vi "Autonomous2Independent.vi"() -> ()   [LabVIEW 2017]
doc: "This VI is called when autonomous begins, and will automatically be terminated when autonomous ends. You can carry out timed or sensor driven robot movement independently without needing to return to the caller."
uses:
  <vilib>/Rock Robotics/WPI/DriverStation/WPI_DriverStationPositionInfo.ctl
  <vilib>/Rock Robotics/WPI/Utilities/WPI_GetSetVariantRefNum.vi
panel:
  out "Distance 32":dbl
  out "Distance 31":dbl
  out "Distance 30":dbl
  out "Distance 29":dbl
  out "Distance 28":dbl
  out "Distance 27":dbl
  out "Distance 26":dbl
  out "Distance 25":dbl
  out "Distance 24":dbl
  out "Distance 23":dbl
  out "Distance 22":dbl
  out "Distance 21":dbl
  out "Distance 20":dbl
  out "Distance 19":dbl
  out "Distance 18":dbl
  out "Distance 17":dbl
  out "Distance 16":dbl
  out "Distance 15":dbl
  out "Distance 14":dbl
  out "Distance 13":dbl
  out "Distance 12":dbl
  out "Distance 11":dbl
  out "Distance 10":dbl
  out "Distance 9":dbl
  out "Distance 6":dbl
  out "Distance 5":dbl
  out "Distance":dbl
  out "Distance 2":dbl
  out "substring":string
  out "Position":T1
  # "Be sure to right-click and choose Data Operations>>Make Current Value default if you want to save the array values with the VI"
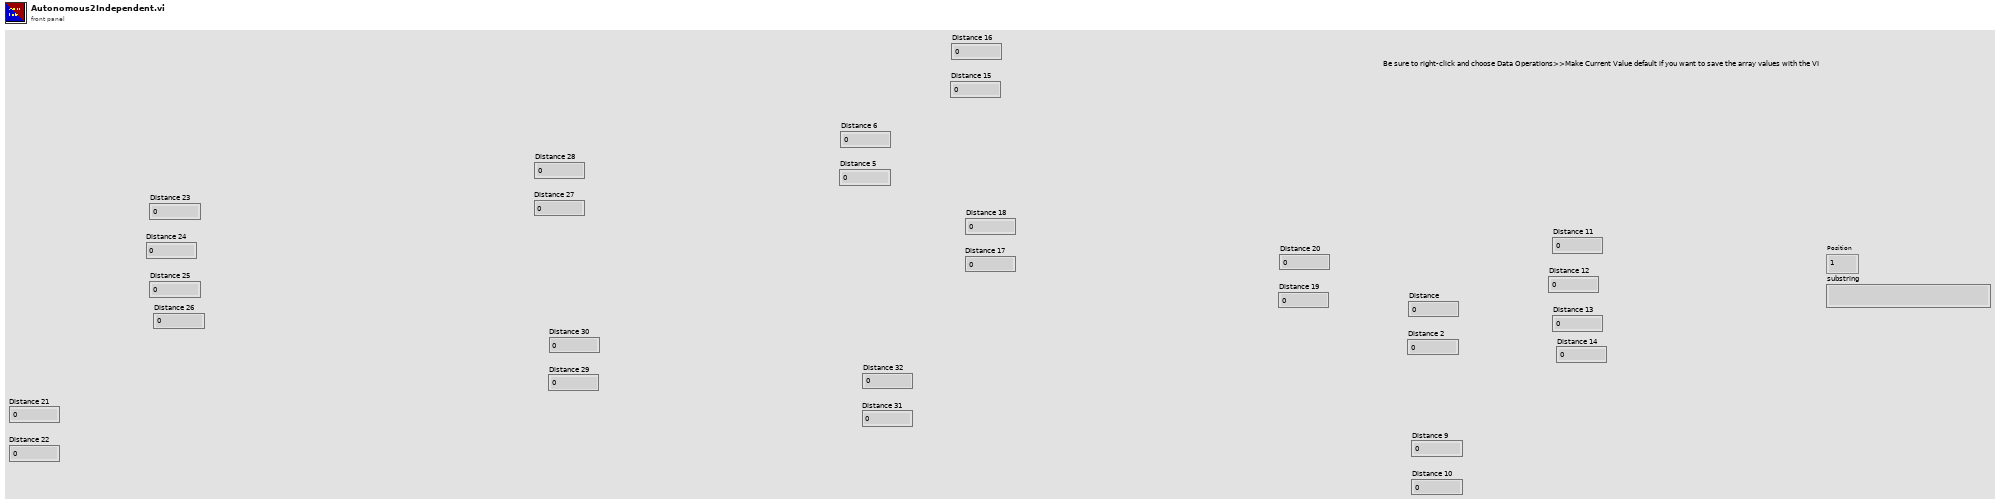
[diagram p1: front panel]
types:
  T1 = typedef "WPI_DriverStationPositionInfo.ctl" = enum16{"1", "2", "3"}
  T2 = typedef "WPI_EncoderDevRef.ctl" = cluster{"DevStatus":errorcluster, "EncoderIndex":T3, "CounterIndex":T4, "DistancePerCount":dbl, "Decoding Type":T5}
  T3 = typedef "FPGA_EncoderIdx.ctl" = enum8{"Enc 0", "Enc 1", "Enc 2", "Enc 3", "Enc 4", "Enc 5", "Enc 6", "Enc 7", "Invalid"}
  T4 = typedef "FPGA_CounterCtrSystemIndex.ctl" = enum8{"Ctr 0", "Ctr 1", "Ctr 2", "Ctr 3", "Ctr 4", "Ctr 5", "Ctr 6", "Ctr 7", "Invalid"}
  T5 = typedef "WPI_EncoderType.ctl" = enum16{"1x", "2x", "4x"}
  T6 = typedef "WPI_RobotDriveDevRef.ctl" = cluster{"DevStatus":errorcluster, "Motors[]":T7[], "Square Inputs":bool, "Max Output":dbl}
  T7 = typedef "WPI_MotorControlDeviceRef.ctl" = cluster{"DeviceStatus":errorcluster, "Type":T8, "PWM":cluster{"PWM Channel":T9, "DeadBand":T10}, "CAN":cluster{"Device Number":u8, "SetOutput VI Ref":variant, "GetOutput VI Ref":variant, "Enable VI Ref":variant, "Disable VI Ref":variant, "Data":variant}, "Invert":bool, "DIO PWM":cluster{"PWM \"Enable\" Channel":T9, "DIOChannel":T11, "PWM Rate":dbl}}
  T8 = typedef "WPI_MotorControlType.ctl" = enum16{"PWM", "CAN", "DIO PWM"}
  T9 = typedef "FPGA_DIOPWMChannel.ctl" = enum8{"PWM 0", "PWM 1", "PWM 2", "PWM 3", "PWM 4", "PWM 5", "PWM 6", "PWM 7", "PWM 8", "PWM 9", "PWM MXP 0", "PWM MXP 1", "PWM MXP 2", "PWM MXP 3", "PWM MXP 4", "PWM MXP 5", "PWM MXP 6", "PWM MXP 7", "PWM MXP 8", "PWM MXP 9", "Invalid"}
  T10 = typedef "WPI_PWMDeadband.ctl" = cluster{"Name":string, "maxPositivePwm":i32, "minPositivePwm":i32, "centerPwm":i32, "maxNegativePwm":i32, "minNegativePwm":i32, "angularRange":u16}
  T11 = typedef "FPGA_DIOChannel.ctl" = enum8{"DIO 0", "DIO 1", "DIO 2", "DIO 3", "DIO 4", "DIO 5", "DIO 6", "DIO 7", "DIO 8", "DIO 9", "DIO MXP 0", "DIO MXP 1", "DIO MXP 2", "DIO MXP 3", "DIO MXP 4", "DIO MXP 5", "DIO MXP 6", "DIO MXP 7", "DIO MXP 8", "DIO MXP 9", "DIO MXP 10", "DIO MXP 11", "DIO MXP 12", "DIO MXP 13", "DIO MXP 14", "DIO MXP 15", "SPI Port CS1", "SPI Port CS2", "SPI Port CS3", "SPI Port MISO", "SPI Port MOSI", "Invalid"}
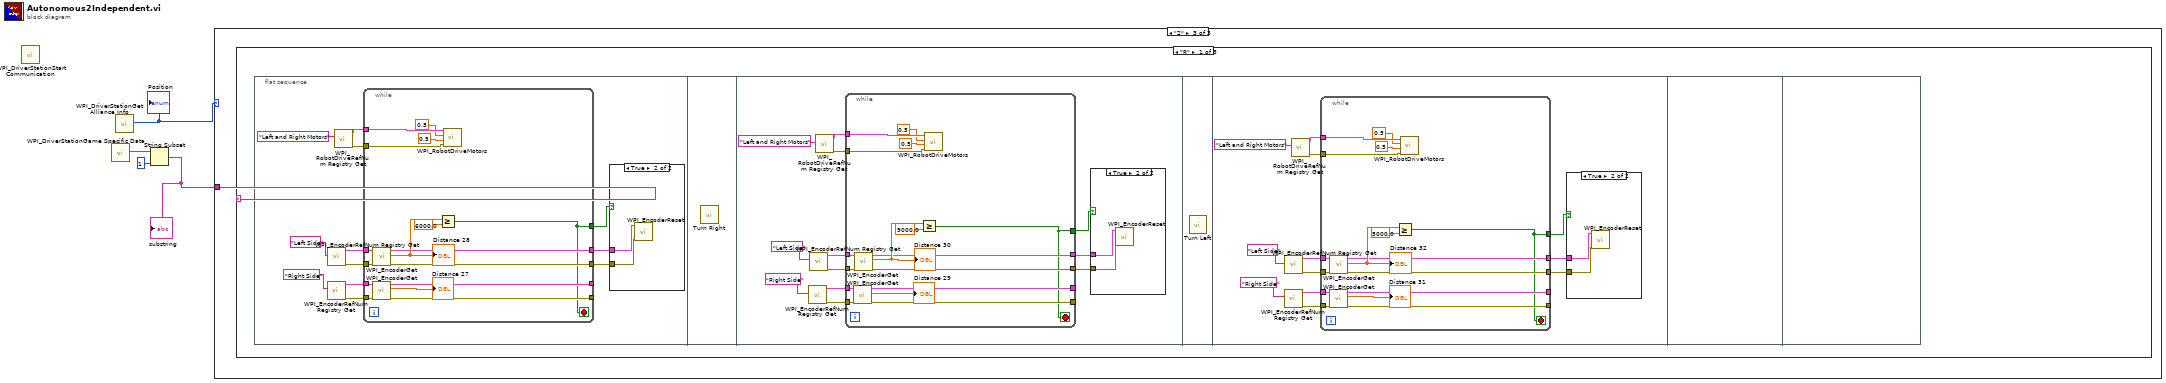
[diagram p0: block diagram]
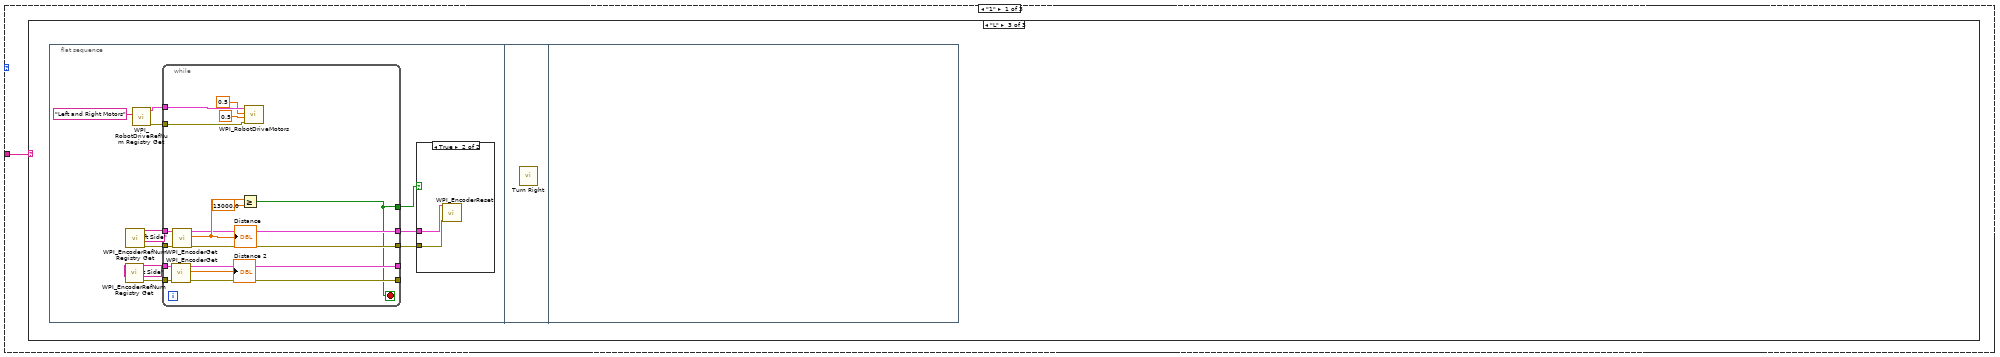
[diagram p2: hidden frame]
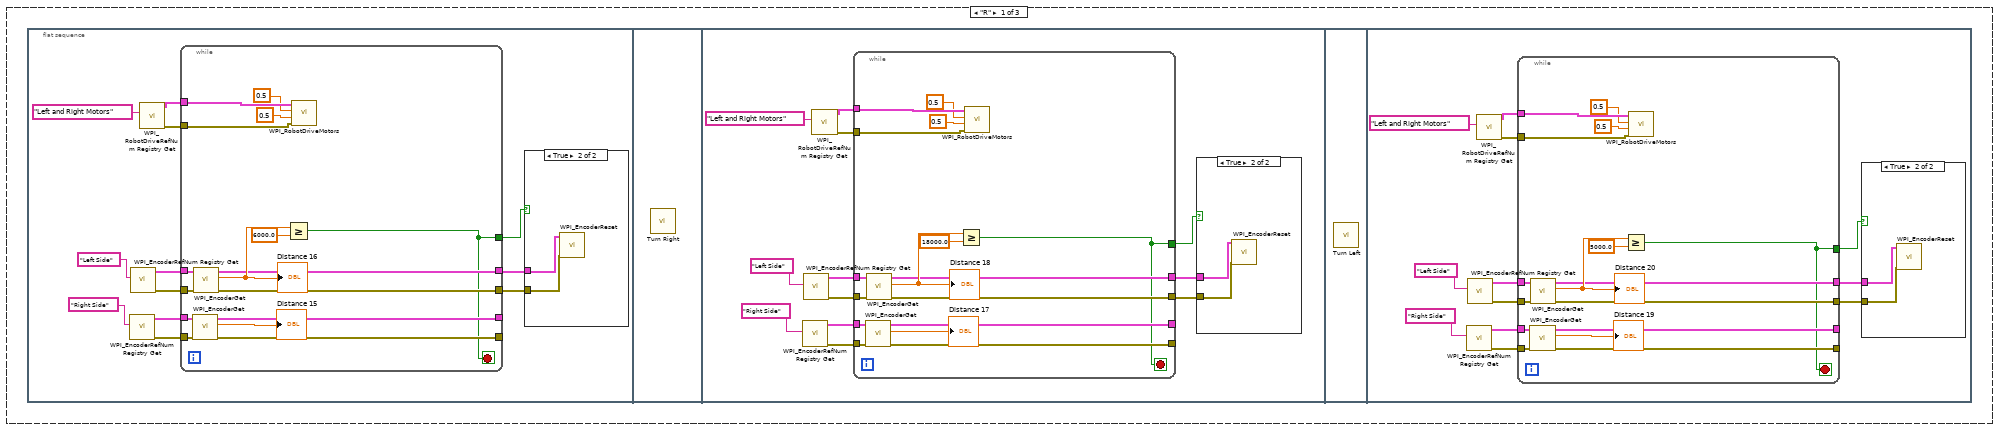
[diagram p3: hidden frame]
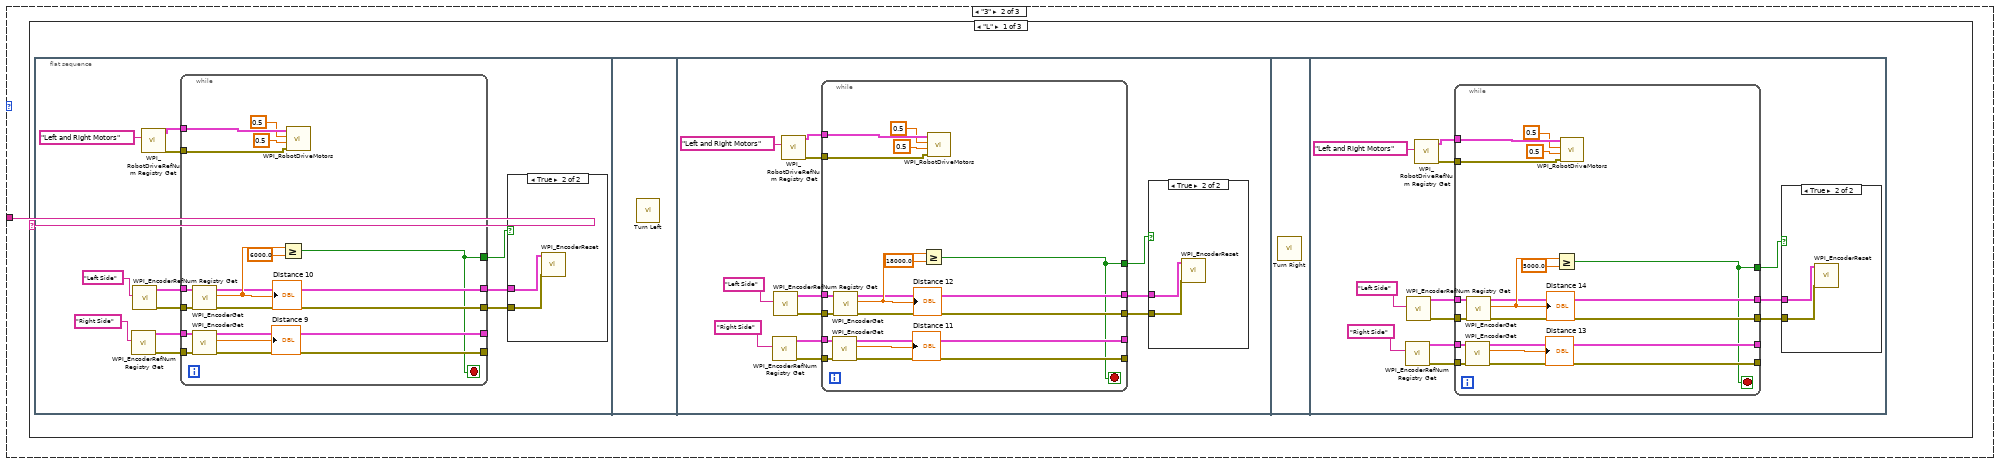
[diagram p9: hidden frame]
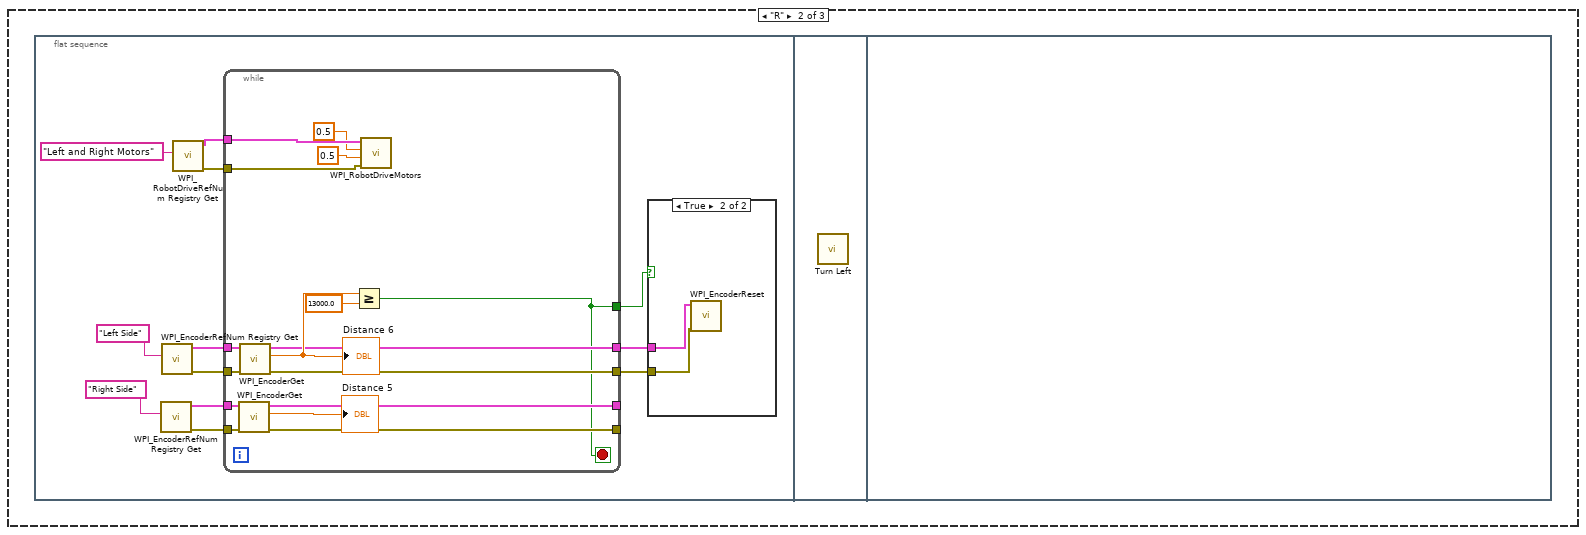
[diagram p13: hidden frame]
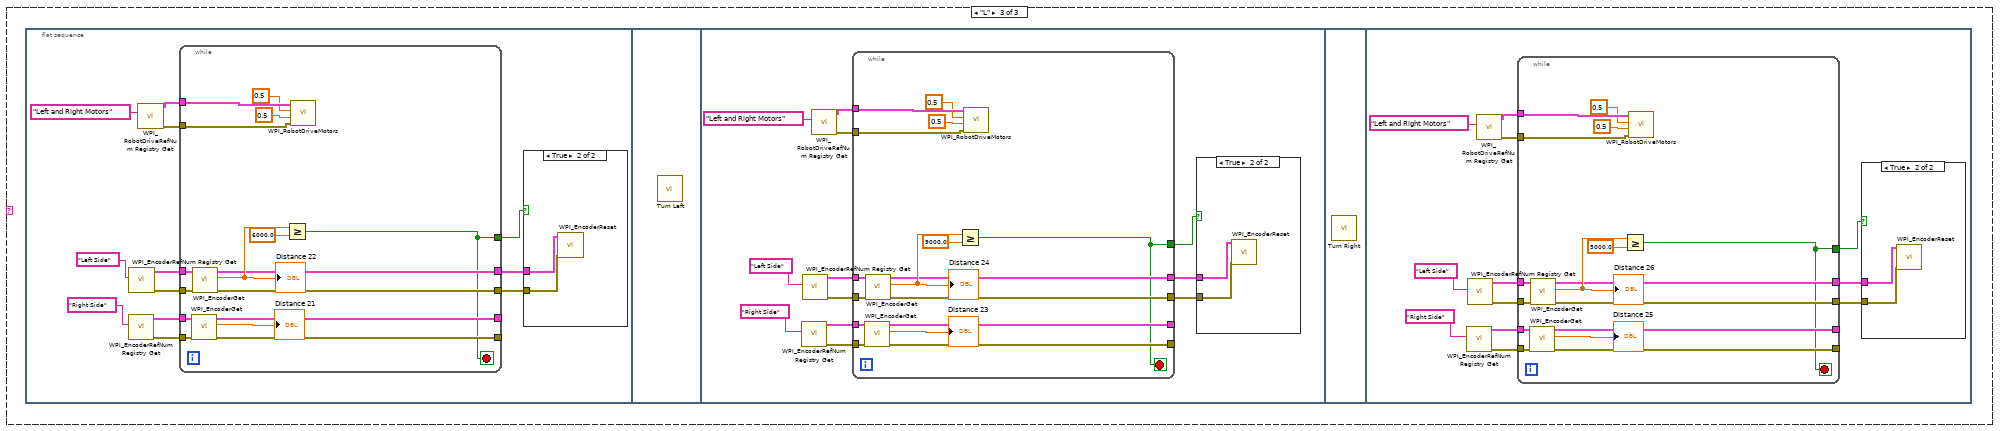
[diagram p20: hidden frame]
diagram:
  n1 = call <vilib>:"WPI_DriverStationStart Communication.vi"() -> ()  [unwired: 12 in]
  n2 = call <vilib>:"WPI_DriverStationGame Specific Data.vi"() -> ("Game Specific Data"=w4:string)  [unwired: 11 in]
  n3 = call <vilib>:"WPI_DriverStationGet Alliance Info.vi"() -> ("Position"=w2:T1)  [unwired: 6 in, 5 out]
  "Position" <- w2
  n4 = String Subset(string=w4, length (rest)=1 ("length (rest)")) -> (substring=w1:string)  [unwired: 1 in]
  "substring" <- w1
  n5 = case shown="\"2\"" w2 {
    tunnel: w1 -> [w5 w126 w247]
    frame "1" {
      n6 = case shown="\"L\"" w5 {
        frame "R" {
          n7 = flat-sequence {
            frame #0 {
              n8 = call <vilib>:"WPI_EncoderRefNum Registry Get.vi"("refnum name"="Right Side") -> ("error out"=w11:errorcluster, "EncoderDevRef"=w12:T2)  [unwired: 9 in]
              n9 = call <vilib>:"WPI_EncoderRefNum Registry Get.vi"("refnum name"="Left Side") -> ("error out"=w10:errorcluster, "EncoderDevRef"=w9:T2)  [unwired: 9 in]
              n10 = call <vilib>:"WPI_RobotDriveRefNum Registry Get.vi"("refnum name"="Left and Right Motors") -> ("error out"=w17:errorcluster, "RobotDriveDevRef"=w16:T6)  [unwired: 9 in]
              n11 = while {
                tunnel: w9 -> [w35]
                tunnel: w10 -> [w34]
                tunnel: w12 -> [w31]
                tunnel: w11 -> [w32]
                tunnel: [w28] -> w14
                tunnel: [w27] -> w15
                tunnel: [w26] -> _
                tunnel: [w25] -> _
                tunnel: [w24] -> w13
                tunnel: w16 -> [w23]
                tunnel: w17 -> [w22]
                stop <- w24 stop-if-true
                n12 = call <vilib>:"WPI_EncoderGet.vi"("error in (no error)"=w32, "EncoderDevRef"=w31) -> ("error out"=w25:errorcluster, "Distance"=→"Distance 15":dbl, "EncoderDevRef"=w26:T2)  [unwired: 4 in, 3 out]
                n13 = call <vilib>:"WPI_EncoderGet.vi"("error in (no error)"=w34, "EncoderDevRef"=w35) -> ("error out"=w27:errorcluster, "Distance"=w30:dbl, "EncoderDevRef"=w28:T2)  [unwired: 4 in, 3 out]
                "Distance 16" <- w30
                n14 = Greater Or Equal?(x=w30, y=6000.0) -> (x >= y?=w24:bool)
                n15 = call <vilib>:"WPI_RobotDriveMotors.vi"("error in (no error)"=w22, "RightSpeed"=0.5, "LeftSpeed"=0.5, "RobotDriveDevRef"=w23) -> ()  [unwired: 5 in, 3 out]
              }
              n16 = case shown="True" w13 {
                tunnel: w14 -> [_ w19]
                tunnel: w15 -> [_ w18]
                frame False {
                }
                frame True {
                  n17 = call <vilib>:"WPI_EncoderReset.vi"("error in (no error)"=w18, "EncoderDevRef"=w19) -> ()  [unwired: 8 in, 2 out]
                }
              }
            }
            frame #1 {
              n18 = call "Turn Right.vi"() -> ()  [unwired: 12 in]
            }
            frame #2 {
              n19 = call <vilib>:"WPI_EncoderRefNum Registry Get.vi"("refnum name"="Right Side") -> ("error out"=w45:errorcluster, "EncoderDevRef"=w44:T2)  [unwired: 9 in]
              n20 = call <vilib>:"WPI_EncoderRefNum Registry Get.vi"("refnum name"="Left Side") -> ("error out"=w46:errorcluster, "EncoderDevRef"=w47:T2)  [unwired: 9 in]
              n21 = call <vilib>:"WPI_RobotDriveRefNum Registry Get.vi"("refnum name"="Left and Right Motors") -> ("error out"=w36:errorcluster, "RobotDriveDevRef"=w37:T6)  [unwired: 9 in]
              n22 = while {
                tunnel: w47 -> [w65]
                tunnel: w46 -> [w64]
                tunnel: w44 -> [w61]
                tunnel: w45 -> [w62]
                tunnel: [w58] -> w40
                tunnel: [w57] -> w39
                tunnel: [w56] -> _
                tunnel: [w55] -> _
                tunnel: [w54] -> w41
                tunnel: w37 -> [w53]
                tunnel: w36 -> [w52]
                stop <- w54 stop-if-true
                n23 = call <vilib>:"WPI_EncoderGet.vi"("error in (no error)"=w62, "EncoderDevRef"=w61) -> ("error out"=w55:errorcluster, "Distance"=→"Distance 17":dbl, "EncoderDevRef"=w56:T2)  [unwired: 4 in, 3 out]
                n24 = call <vilib>:"WPI_EncoderGet.vi"("error in (no error)"=w64, "EncoderDevRef"=w65) -> ("error out"=w57:errorcluster, "Distance"=w60:dbl, "EncoderDevRef"=w58:T2)  [unwired: 4 in, 3 out]
                "Distance 18" <- w60
                n25 = Greater Or Equal?(x=w60, y=18000.0) -> (x >= y?=w54:bool)
                n26 = call <vilib>:"WPI_RobotDriveMotors.vi"("error in (no error)"=w52, "RightSpeed"=0.5, "LeftSpeed"=0.5, "RobotDriveDevRef"=w53) -> ()  [unwired: 5 in, 3 out]
              }
              n27 = case shown="True" w41 {
                tunnel: w40 -> [_ w49]
                tunnel: w39 -> [_ w48]
                frame False {
                }
                frame True {
                  n28 = call <vilib>:"WPI_EncoderReset.vi"("error in (no error)"=w48, "EncoderDevRef"=w49) -> ()  [unwired: 8 in, 2 out]
                }
              }
            }
            frame #3 {
              n29 = call "Turn Left.vi"() -> ()  [unwired: 12 in]
            }
            frame #4 {
              n30 = call <vilib>:"WPI_EncoderRefNum Registry Get.vi"("refnum name"="Right Side") -> ("error out"=w75:errorcluster, "EncoderDevRef"=w74:T2)  [unwired: 9 in]
              n31 = call <vilib>:"WPI_EncoderRefNum Registry Get.vi"("refnum name"="Left Side") -> ("error out"=w76:errorcluster, "EncoderDevRef"=w77:T2)  [unwired: 9 in]
              n32 = call <vilib>:"WPI_RobotDriveRefNum Registry Get.vi"("refnum name"="Left and Right Motors") -> ("error out"=w66:errorcluster, "RobotDriveDevRef"=w67:T6)  [unwired: 9 in]
              n33 = while {
                tunnel: w77 -> [w95]
                tunnel: w76 -> [w94]
                tunnel: w74 -> [w91]
                tunnel: w75 -> [w92]
                tunnel: [w88] -> w70
                tunnel: [w87] -> w69
                tunnel: [w86] -> _
                tunnel: [w85] -> _
                tunnel: [w84] -> w71
                tunnel: w67 -> [w83]
                tunnel: w66 -> [w82]
                stop <- w84 stop-if-true
                n34 = call <vilib>:"WPI_EncoderGet.vi"("error in (no error)"=w92, "EncoderDevRef"=w91) -> ("error out"=w85:errorcluster, "Distance"=→"Distance 19":dbl, "EncoderDevRef"=w86:T2)  [unwired: 4 in, 3 out]
                n35 = call <vilib>:"WPI_EncoderGet.vi"("error in (no error)"=w94, "EncoderDevRef"=w95) -> ("error out"=w87:errorcluster, "Distance"=w90:dbl, "EncoderDevRef"=w88:T2)  [unwired: 4 in, 3 out]
                "Distance 20" <- w90
                n36 = Greater Or Equal?(x=w90, y=5000.0) -> (x >= y?=w84:bool)
                n37 = call <vilib>:"WPI_RobotDriveMotors.vi"("error in (no error)"=w82, "RightSpeed"=0.5, "LeftSpeed"=0.5, "RobotDriveDevRef"=w83) -> ()  [unwired: 5 in, 3 out]
              }
              n38 = case shown="True" w71 {
                tunnel: w70 -> [_ w79]
                tunnel: w69 -> [_ w78]
                frame False {
                }
                frame True {
                  n39 = call <vilib>:"WPI_EncoderReset.vi"("error in (no error)"=w78, "EncoderDevRef"=w79) -> ()  [unwired: 8 in, 2 out]
                }
              }
            }
          }
        }
        frame Default {
        }
        frame "L" {
          n40 = flat-sequence {
            frame #0 {
              n41 = call <vilib>:"WPI_EncoderRefNum Registry Get.vi"("refnum name"="Right Side") -> ("error out"=w105:errorcluster, "EncoderDevRef"=w104:T2)  [unwired: 9 in]
              n42 = call <vilib>:"WPI_EncoderRefNum Registry Get.vi"("refnum name"="Left Side") -> ("error out"=w106:errorcluster, "EncoderDevRef"=w107:T2)  [unwired: 9 in]
              n43 = call <vilib>:"WPI_RobotDriveRefNum Registry Get.vi"("refnum name"="Left and Right Motors") -> ("error out"=w96:errorcluster, "RobotDriveDevRef"=w97:T6)  [unwired: 9 in]
              n44 = while {
                tunnel: w107 -> [w125]
                tunnel: w106 -> [w124]
                tunnel: w104 -> [w121]
                tunnel: w105 -> [w122]
                tunnel: [w118] -> w100
                tunnel: [w117] -> w99
                tunnel: [w116] -> _
                tunnel: [w115] -> _
                tunnel: [w114] -> w101
                tunnel: w97 -> [w113]
                tunnel: w96 -> [w112]
                stop <- w114 stop-if-true
                n45 = call <vilib>:"WPI_EncoderGet.vi"("error in (no error)"=w122, "EncoderDevRef"=w121) -> ("error out"=w115:errorcluster, "Distance"=→"Distance 2":dbl, "EncoderDevRef"=w116:T2)  [unwired: 4 in, 3 out]
                n46 = call <vilib>:"WPI_EncoderGet.vi"("error in (no error)"=w124, "EncoderDevRef"=w125) -> ("error out"=w117:errorcluster, "Distance"=w120:dbl, "EncoderDevRef"=w118:T2)  [unwired: 4 in, 3 out]
                "Distance" <- w120
                n47 = Greater Or Equal?(x=w120, y=13000.0) -> (x >= y?=w114:bool)
                n48 = call <vilib>:"WPI_RobotDriveMotors.vi"("error in (no error)"=w112, "RightSpeed"=0.5, "LeftSpeed"=0.5, "RobotDriveDevRef"=w113) -> ()  [unwired: 5 in, 3 out]
              }
              n49 = case shown="True" w101 {
                tunnel: w100 -> [_ w109]
                tunnel: w99 -> [_ w108]
                frame False {
                }
                frame True {
                  n50 = call <vilib>:"WPI_EncoderReset.vi"("error in (no error)"=w108, "EncoderDevRef"=w109) -> ()  [unwired: 8 in, 2 out]
                }
              }
            }
            frame #1 {
              n51 = call "Turn Right.vi"() -> ()  [unwired: 12 in]
            }
            frame #2 {
            }
          }
        }
      }
    }
    frame "3" {
      n52 = case shown="\"L\"" w126 {
        frame "L" {
          n53 = flat-sequence {
            frame #0 {
              n54 = call <vilib>:"WPI_EncoderRefNum Registry Get.vi"("refnum name"="Right Side") -> ("error out"=w132:errorcluster, "EncoderDevRef"=w133:T2)  [unwired: 9 in]
              n55 = call <vilib>:"WPI_EncoderRefNum Registry Get.vi"("refnum name"="Left Side") -> ("error out"=w131:errorcluster, "EncoderDevRef"=w130:T2)  [unwired: 9 in]
              n56 = call <vilib>:"WPI_RobotDriveRefNum Registry Get.vi"("refnum name"="Left and Right Motors") -> ("error out"=w138:errorcluster, "RobotDriveDevRef"=w137:T6)  [unwired: 9 in]
              n57 = while {
                tunnel: w130 -> [w156]
                tunnel: w131 -> [w155]
                tunnel: w133 -> [w152]
                tunnel: w132 -> [w153]
                tunnel: [w149] -> w135
                tunnel: [w148] -> w136
                tunnel: [w147] -> _
                tunnel: [w146] -> _
                tunnel: [w145] -> w134
                tunnel: w137 -> [w144]
                tunnel: w138 -> [w143]
                stop <- w145 stop-if-true
                n58 = call <vilib>:"WPI_EncoderGet.vi"("error in (no error)"=w153, "EncoderDevRef"=w152) -> ("error out"=w146:errorcluster, "Distance"=→"Distance 9":dbl, "EncoderDevRef"=w147:T2)  [unwired: 4 in, 3 out]
                n59 = call <vilib>:"WPI_EncoderGet.vi"("error in (no error)"=w155, "EncoderDevRef"=w156) -> ("error out"=w148:errorcluster, "Distance"=w151:dbl, "EncoderDevRef"=w149:T2)  [unwired: 4 in, 3 out]
                "Distance 10" <- w151
                n60 = Greater Or Equal?(x=w151, y=6000.0) -> (x >= y?=w145:bool)
                n61 = call <vilib>:"WPI_RobotDriveMotors.vi"("error in (no error)"=w143, "RightSpeed"=0.5, "LeftSpeed"=0.5, "RobotDriveDevRef"=w144) -> ()  [unwired: 5 in, 3 out]
              }
              n62 = case shown="True" w134 {
                tunnel: w135 -> [_ w140]
                tunnel: w136 -> [_ w139]
                frame False {
                }
                frame True {
                  n63 = call <vilib>:"WPI_EncoderReset.vi"("error in (no error)"=w139, "EncoderDevRef"=w140) -> ()  [unwired: 8 in, 2 out]
                }
              }
            }
            frame #1 {
              n64 = call "Turn Left.vi"() -> ()  [unwired: 12 in]
            }
            frame #2 {
              n65 = call <vilib>:"WPI_EncoderRefNum Registry Get.vi"("refnum name"="Right Side") -> ("error out"=w166:errorcluster, "EncoderDevRef"=w165:T2)  [unwired: 9 in]
              n66 = call <vilib>:"WPI_EncoderRefNum Registry Get.vi"("refnum name"="Left Side") -> ("error out"=w167:errorcluster, "EncoderDevRef"=w168:T2)  [unwired: 9 in]
              n67 = call <vilib>:"WPI_RobotDriveRefNum Registry Get.vi"("refnum name"="Left and Right Motors") -> ("error out"=w157:errorcluster, "RobotDriveDevRef"=w158:T6)  [unwired: 9 in]
              n68 = while {
                tunnel: w168 -> [w186]
                tunnel: w167 -> [w185]
                tunnel: w165 -> [w182]
                tunnel: w166 -> [w183]
                tunnel: [w179] -> w161
                tunnel: [w178] -> w160
                tunnel: [w177] -> _
                tunnel: [w176] -> _
                tunnel: [w175] -> w162
                tunnel: w158 -> [w174]
                tunnel: w157 -> [w173]
                stop <- w175 stop-if-true
                n69 = call <vilib>:"WPI_EncoderGet.vi"("error in (no error)"=w183, "EncoderDevRef"=w182) -> ("error out"=w176:errorcluster, "Distance"=→"Distance 11":dbl, "EncoderDevRef"=w177:T2)  [unwired: 4 in, 3 out]
                n70 = call <vilib>:"WPI_EncoderGet.vi"("error in (no error)"=w185, "EncoderDevRef"=w186) -> ("error out"=w178:errorcluster, "Distance"=w181:dbl, "EncoderDevRef"=w179:T2)  [unwired: 4 in, 3 out]
                "Distance 12" <- w181
                n71 = Greater Or Equal?(x=w181, y=18000.0) -> (x >= y?=w175:bool)
                n72 = call <vilib>:"WPI_RobotDriveMotors.vi"("error in (no error)"=w173, "RightSpeed"=0.5, "LeftSpeed"=0.5, "RobotDriveDevRef"=w174) -> ()  [unwired: 5 in, 3 out]
              }
              n73 = case shown="True" w162 {
                tunnel: w161 -> [_ w170]
                tunnel: w160 -> [_ w169]
                frame False {
                }
                frame True {
                  n74 = call <vilib>:"WPI_EncoderReset.vi"("error in (no error)"=w169, "EncoderDevRef"=w170) -> ()  [unwired: 8 in, 2 out]
                }
              }
            }
            frame #3 {
              n75 = call "Turn Right.vi"() -> ()  [unwired: 12 in]
            }
            frame #4 {
              n76 = call <vilib>:"WPI_EncoderRefNum Registry Get.vi"("refnum name"="Right Side") -> ("error out"=w196:errorcluster, "EncoderDevRef"=w195:T2)  [unwired: 9 in]
              n77 = call <vilib>:"WPI_EncoderRefNum Registry Get.vi"("refnum name"="Left Side") -> ("error out"=w197:errorcluster, "EncoderDevRef"=w198:T2)  [unwired: 9 in]
              n78 = call <vilib>:"WPI_RobotDriveRefNum Registry Get.vi"("refnum name"="Left and Right Motors") -> ("error out"=w187:errorcluster, "RobotDriveDevRef"=w188:T6)  [unwired: 9 in]
              n79 = while {
                tunnel: w198 -> [w216]
                tunnel: w197 -> [w215]
                tunnel: w195 -> [w212]
                tunnel: w196 -> [w213]
                tunnel: [w209] -> w191
                tunnel: [w208] -> w190
                tunnel: [w207] -> _
                tunnel: [w206] -> _
                tunnel: [w205] -> w192
                tunnel: w188 -> [w204]
                tunnel: w187 -> [w203]
                stop <- w205 stop-if-true
                n80 = call <vilib>:"WPI_EncoderGet.vi"("error in (no error)"=w213, "EncoderDevRef"=w212) -> ("error out"=w206:errorcluster, "Distance"=→"Distance 13":dbl, "EncoderDevRef"=w207:T2)  [unwired: 4 in, 3 out]
                n81 = call <vilib>:"WPI_EncoderGet.vi"("error in (no error)"=w215, "EncoderDevRef"=w216) -> ("error out"=w208:errorcluster, "Distance"=w211:dbl, "EncoderDevRef"=w209:T2)  [unwired: 4 in, 3 out]
                "Distance 14" <- w211
                n82 = Greater Or Equal?(x=w211, y=5000.0) -> (x >= y?=w205:bool)
                n83 = call <vilib>:"WPI_RobotDriveMotors.vi"("error in (no error)"=w203, "RightSpeed"=0.5, "LeftSpeed"=0.5, "RobotDriveDevRef"=w204) -> ()  [unwired: 5 in, 3 out]
              }
              n84 = case shown="True" w192 {
                tunnel: w191 -> [_ w200]
                tunnel: w190 -> [_ w199]
                frame False {
                }
                frame True {
                  n85 = call <vilib>:"WPI_EncoderReset.vi"("error in (no error)"=w199, "EncoderDevRef"=w200) -> ()  [unwired: 8 in, 2 out]
                }
              }
            }
          }
        }
        frame "R" {
          n86 = flat-sequence {
            frame #0 {
              n87 = call <vilib>:"WPI_EncoderRefNum Registry Get.vi"("refnum name"="Right Side") -> ("error out"=w226:errorcluster, "EncoderDevRef"=w225:T2)  [unwired: 9 in]
              n88 = call <vilib>:"WPI_EncoderRefNum Registry Get.vi"("refnum name"="Left Side") -> ("error out"=w227:errorcluster, "EncoderDevRef"=w228:T2)  [unwired: 9 in]
              n89 = call <vilib>:"WPI_RobotDriveRefNum Registry Get.vi"("refnum name"="Left and Right Motors") -> ("error out"=w217:errorcluster, "RobotDriveDevRef"=w218:T6)  [unwired: 9 in]
              n90 = while {
                tunnel: w228 -> [w246]
                tunnel: w227 -> [w245]
                tunnel: w225 -> [w242]
                tunnel: w226 -> [w243]
                tunnel: [w239] -> w221
                tunnel: [w238] -> w220
                tunnel: [w237] -> _
                tunnel: [w236] -> _
                tunnel: [w235] -> w222
                tunnel: w218 -> [w234]
                tunnel: w217 -> [w233]
                stop <- w235 stop-if-true
                n91 = call <vilib>:"WPI_EncoderGet.vi"("error in (no error)"=w243, "EncoderDevRef"=w242) -> ("error out"=w236:errorcluster, "Distance"=→"Distance 5":dbl, "EncoderDevRef"=w237:T2)  [unwired: 4 in, 3 out]
                n92 = call <vilib>:"WPI_EncoderGet.vi"("error in (no error)"=w245, "EncoderDevRef"=w246) -> ("error out"=w238:errorcluster, "Distance"=w241:dbl, "EncoderDevRef"=w239:T2)  [unwired: 4 in, 3 out]
                "Distance 6" <- w241
                n93 = Greater Or Equal?(x=w241, y=13000.0) -> (x >= y?=w235:bool)
                n94 = call <vilib>:"WPI_RobotDriveMotors.vi"("error in (no error)"=w233, "RightSpeed"=0.5, "LeftSpeed"=0.5, "RobotDriveDevRef"=w234) -> ()  [unwired: 5 in, 3 out]
              }
              n95 = case shown="True" w222 {
                tunnel: w221 -> [_ w230]
                tunnel: w220 -> [_ w229]
                frame False {
                }
                frame True {
                  n96 = call <vilib>:"WPI_EncoderReset.vi"("error in (no error)"=w229, "EncoderDevRef"=w230) -> ()  [unwired: 8 in, 2 out]
                }
              }
            }
            frame #1 {
              n97 = call "Turn Left.vi"() -> ()  [unwired: 12 in]
            }
            frame #2 {
            }
          }
        }
        frame Default {
        }
      }
    }
    frame "2" {
      n98 = case shown="\"R\"" w247 {
        frame "R" {
          n99 = flat-sequence {
            frame #0 {
              n100 = call <vilib>:"WPI_EncoderRefNum Registry Get.vi"("refnum name"="Right Side") -> ("error out"=w253:errorcluster, "EncoderDevRef"=w254:T2)  [unwired: 9 in]
              n101 = call <vilib>:"WPI_EncoderRefNum Registry Get.vi"("refnum name"="Left Side") -> ("error out"=w252:errorcluster, "EncoderDevRef"=w251:T2)  [unwired: 9 in]
              n102 = call <vilib>:"WPI_RobotDriveRefNum Registry Get.vi"("refnum name"="Left and Right Motors") -> ("error out"=w259:errorcluster, "RobotDriveDevRef"=w258:T6)  [unwired: 9 in]
              n103 = while {
                tunnel: w251 -> [w277]
                tunnel: w252 -> [w276]
                tunnel: w254 -> [w273]
                tunnel: w253 -> [w274]
                tunnel: [w270] -> w256
                tunnel: [w269] -> w257
                tunnel: [w268] -> _
                tunnel: [w267] -> _
                tunnel: [w266] -> w255
                tunnel: w258 -> [w265]
                tunnel: w259 -> [w264]
                stop <- w266 stop-if-true
                n104 = call <vilib>:"WPI_EncoderGet.vi"("error in (no error)"=w274, "EncoderDevRef"=w273) -> ("error out"=w267:errorcluster, "Distance"=→"Distance 27":dbl, "EncoderDevRef"=w268:T2)  [unwired: 4 in, 3 out]
                n105 = call <vilib>:"WPI_EncoderGet.vi"("error in (no error)"=w276, "EncoderDevRef"=w277) -> ("error out"=w269:errorcluster, "Distance"=w272:dbl, "EncoderDevRef"=w270:T2)  [unwired: 4 in, 3 out]
                "Distance 28" <- w272
                n106 = Greater Or Equal?(x=w272, y=6000.0) -> (x >= y?=w266:bool)
                n107 = call <vilib>:"WPI_RobotDriveMotors.vi"("error in (no error)"=w264, "RightSpeed"=0.5, "LeftSpeed"=0.5, "RobotDriveDevRef"=w265) -> ()  [unwired: 5 in, 3 out]
              }
              n108 = case shown="True" w255 {
                tunnel: w256 -> [_ w261]
                tunnel: w257 -> [_ w260]
                frame False {
                }
                frame True {
                  n109 = call <vilib>:"WPI_EncoderReset.vi"("error in (no error)"=w260, "EncoderDevRef"=w261) -> ()  [unwired: 8 in, 2 out]
                }
              }
            }
            frame #1 {
              n110 = call "Turn Right.vi"() -> ()  [unwired: 12 in]
            }
            frame #2 {
              n111 = call <vilib>:"WPI_EncoderRefNum Registry Get.vi"("refnum name"="Right Side") -> ("error out"=w287:errorcluster, "EncoderDevRef"=w286:T2)  [unwired: 9 in]
              n112 = call <vilib>:"WPI_EncoderRefNum Registry Get.vi"("refnum name"="Left Side") -> ("error out"=w288:errorcluster, "EncoderDevRef"=w289:T2)  [unwired: 9 in]
              n113 = call <vilib>:"WPI_RobotDriveRefNum Registry Get.vi"("refnum name"="Left and Right Motors") -> ("error out"=w278:errorcluster, "RobotDriveDevRef"=w279:T6)  [unwired: 9 in]
              n114 = while {
                tunnel: w289 -> [w307]
                tunnel: w288 -> [w306]
                tunnel: w286 -> [w303]
                tunnel: w287 -> [w304]
                tunnel: [w300] -> w282
                tunnel: [w299] -> w281
                tunnel: [w298] -> _
                tunnel: [w297] -> _
                tunnel: [w296] -> w283
                tunnel: w279 -> [w295]
                tunnel: w278 -> [w294]
                stop <- w296 stop-if-true
                n115 = call <vilib>:"WPI_EncoderGet.vi"("error in (no error)"=w304, "EncoderDevRef"=w303) -> ("error out"=w297:errorcluster, "Distance"=→"Distance 29":dbl, "EncoderDevRef"=w298:T2)  [unwired: 4 in, 3 out]
                n116 = call <vilib>:"WPI_EncoderGet.vi"("error in (no error)"=w306, "EncoderDevRef"=w307) -> ("error out"=w299:errorcluster, "Distance"=w302:dbl, "EncoderDevRef"=w300:T2)  [unwired: 4 in, 3 out]
                "Distance 30" <- w302
                n117 = Greater Or Equal?(x=w302, y=9000.0) -> (x >= y?=w296:bool)
                n118 = call <vilib>:"WPI_RobotDriveMotors.vi"("error in (no error)"=w294, "RightSpeed"=0.5, "LeftSpeed"=0.5, "RobotDriveDevRef"=w295) -> ()  [unwired: 5 in, 3 out]
              }
              n119 = case shown="True" w283 {
                tunnel: w282 -> [_ w291]
                tunnel: w281 -> [_ w290]
                frame False {
                }
                frame True {
                  n120 = call <vilib>:"WPI_EncoderReset.vi"("error in (no error)"=w290, "EncoderDevRef"=w291) -> ()  [unwired: 8 in, 2 out]
                }
              }
            }
            frame #3 {
              n121 = call "Turn Left.vi"() -> ()  [unwired: 12 in]
            }
            frame #4 {
              n122 = call <vilib>:"WPI_EncoderRefNum Registry Get.vi"("refnum name"="Right Side") -> ("error out"=w317:errorcluster, "EncoderDevRef"=w316:T2)  [unwired: 9 in]
              n123 = call <vilib>:"WPI_EncoderRefNum Registry Get.vi"("refnum name"="Left Side") -> ("error out"=w318:errorcluster, "EncoderDevRef"=w319:T2)  [unwired: 9 in]
              n124 = call <vilib>:"WPI_RobotDriveRefNum Registry Get.vi"("refnum name"="Left and Right Motors") -> ("error out"=w308:errorcluster, "RobotDriveDevRef"=w309:T6)  [unwired: 9 in]
              n125 = while {
                tunnel: w319 -> [w337]
                tunnel: w318 -> [w336]
                tunnel: w316 -> [w333]
                tunnel: w317 -> [w334]
                tunnel: [w330] -> w312
                tunnel: [w329] -> w311
                tunnel: [w328] -> _
                tunnel: [w327] -> _
                tunnel: [w326] -> w313
                tunnel: w309 -> [w325]
                tunnel: w308 -> [w324]
                stop <- w326 stop-if-true
                n126 = call <vilib>:"WPI_EncoderGet.vi"("error in (no error)"=w334, "EncoderDevRef"=w333) -> ("error out"=w327:errorcluster, "Distance"=→"Distance 31":dbl, "EncoderDevRef"=w328:T2)  [unwired: 4 in, 3 out]
                n127 = call <vilib>:"WPI_EncoderGet.vi"("error in (no error)"=w336, "EncoderDevRef"=w337) -> ("error out"=w329:errorcluster, "Distance"=w332:dbl, "EncoderDevRef"=w330:T2)  [unwired: 4 in, 3 out]
                "Distance 32" <- w332
                n128 = Greater Or Equal?(x=w332, y=5000.0) -> (x >= y?=w326:bool)
                n129 = call <vilib>:"WPI_RobotDriveMotors.vi"("error in (no error)"=w324, "RightSpeed"=0.5, "LeftSpeed"=0.5, "RobotDriveDevRef"=w325) -> ()  [unwired: 5 in, 3 out]
              }
              n130 = case shown="True" w313 {
                tunnel: w312 -> [_ w321]
                tunnel: w311 -> [_ w320]
                frame False {
                }
                frame True {
                  n131 = call <vilib>:"WPI_EncoderReset.vi"("error in (no error)"=w320, "EncoderDevRef"=w321) -> ()  [unwired: 8 in, 2 out]
                }
              }
            }
            frame #5 {
            }
            frame #6 {
            }
          }
        }
        frame Default {
        }
        frame "L" {
          n132 = flat-sequence {
            frame #0 {
              n133 = call <vilib>:"WPI_EncoderRefNum Registry Get.vi"("refnum name"="Right Side") -> ("error out"=w343:errorcluster, "EncoderDevRef"=w344:T2)  [unwired: 9 in]
              n134 = call <vilib>:"WPI_EncoderRefNum Registry Get.vi"("refnum name"="Left Side") -> ("error out"=w342:errorcluster, "EncoderDevRef"=w341:T2)  [unwired: 9 in]
              n135 = call <vilib>:"WPI_RobotDriveRefNum Registry Get.vi"("refnum name"="Left and Right Motors") -> ("error out"=w349:errorcluster, "RobotDriveDevRef"=w348:T6)  [unwired: 9 in]
              n136 = while {
                tunnel: w341 -> [w367]
                tunnel: w342 -> [w366]
                tunnel: w344 -> [w363]
                tunnel: w343 -> [w364]
                tunnel: [w360] -> w346
                tunnel: [w359] -> w347
                tunnel: [w358] -> _
                tunnel: [w357] -> _
                tunnel: [w356] -> w345
                tunnel: w348 -> [w355]
                tunnel: w349 -> [w354]
                stop <- w356 stop-if-true
                n137 = call <vilib>:"WPI_EncoderGet.vi"("error in (no error)"=w364, "EncoderDevRef"=w363) -> ("error out"=w357:errorcluster, "Distance"=→"Distance 21":dbl, "EncoderDevRef"=w358:T2)  [unwired: 4 in, 3 out]
                n138 = call <vilib>:"WPI_EncoderGet.vi"("error in (no error)"=w366, "EncoderDevRef"=w367) -> ("error out"=w359:errorcluster, "Distance"=w362:dbl, "EncoderDevRef"=w360:T2)  [unwired: 4 in, 3 out]
                "Distance 22" <- w362
                n139 = Greater Or Equal?(x=w362, y=6000.0) -> (x >= y?=w356:bool)
                n140 = call <vilib>:"WPI_RobotDriveMotors.vi"("error in (no error)"=w354, "RightSpeed"=0.5, "LeftSpeed"=0.5, "RobotDriveDevRef"=w355) -> ()  [unwired: 5 in, 3 out]
              }
              n141 = case shown="True" w345 {
                tunnel: w346 -> [_ w351]
                tunnel: w347 -> [_ w350]
                frame False {
                }
                frame True {
                  n142 = call <vilib>:"WPI_EncoderReset.vi"("error in (no error)"=w350, "EncoderDevRef"=w351) -> ()  [unwired: 8 in, 2 out]
                }
              }
            }
            frame #1 {
              n143 = call "Turn Left.vi"() -> ()  [unwired: 12 in]
            }
            frame #2 {
              n144 = call <vilib>:"WPI_EncoderRefNum Registry Get.vi"("refnum name"="Right Side") -> ("error out"=w377:errorcluster, "EncoderDevRef"=w376:T2)  [unwired: 9 in]
              n145 = call <vilib>:"WPI_EncoderRefNum Registry Get.vi"("refnum name"="Left Side") -> ("error out"=w378:errorcluster, "EncoderDevRef"=w379:T2)  [unwired: 9 in]
              n146 = call <vilib>:"WPI_RobotDriveRefNum Registry Get.vi"("refnum name"="Left and Right Motors") -> ("error out"=w368:errorcluster, "RobotDriveDevRef"=w369:T6)  [unwired: 9 in]
              n147 = while {
                tunnel: w379 -> [w397]
                tunnel: w378 -> [w396]
                tunnel: w376 -> [w393]
                tunnel: w377 -> [w394]
                tunnel: [w390] -> w372
                tunnel: [w389] -> w371
                tunnel: [w388] -> _
                tunnel: [w387] -> _
                tunnel: [w386] -> w373
                tunnel: w369 -> [w385]
                tunnel: w368 -> [w384]
                stop <- w386 stop-if-true
                n148 = call <vilib>:"WPI_EncoderGet.vi"("error in (no error)"=w394, "EncoderDevRef"=w393) -> ("error out"=w387:errorcluster, "Distance"=→"Distance 23":dbl, "EncoderDevRef"=w388:T2)  [unwired: 4 in, 3 out]
                n149 = call <vilib>:"WPI_EncoderGet.vi"("error in (no error)"=w396, "EncoderDevRef"=w397) -> ("error out"=w389:errorcluster, "Distance"=w392:dbl, "EncoderDevRef"=w390:T2)  [unwired: 4 in, 3 out]
                "Distance 24" <- w392
                n150 = Greater Or Equal?(x=w392, y=9000.0) -> (x >= y?=w386:bool)
                n151 = call <vilib>:"WPI_RobotDriveMotors.vi"("error in (no error)"=w384, "RightSpeed"=0.5, "LeftSpeed"=0.5, "RobotDriveDevRef"=w385) -> ()  [unwired: 5 in, 3 out]
              }
              n152 = case shown="True" w373 {
                tunnel: w372 -> [_ w381]
                tunnel: w371 -> [_ w380]
                frame False {
                }
                frame True {
                  n153 = call <vilib>:"WPI_EncoderReset.vi"("error in (no error)"=w380, "EncoderDevRef"=w381) -> ()  [unwired: 8 in, 2 out]
                }
              }
            }
            frame #3 {
              n154 = call "Turn Right.vi"() -> ()  [unwired: 12 in]
            }
            frame #4 {
              n155 = call <vilib>:"WPI_EncoderRefNum Registry Get.vi"("refnum name"="Right Side") -> ("error out"=w407:errorcluster, "EncoderDevRef"=w406:T2)  [unwired: 9 in]
              n156 = call <vilib>:"WPI_EncoderRefNum Registry Get.vi"("refnum name"="Left Side") -> ("error out"=w408:errorcluster, "EncoderDevRef"=w409:T2)  [unwired: 9 in]
              n157 = call <vilib>:"WPI_RobotDriveRefNum Registry Get.vi"("refnum name"="Left and Right Motors") -> ("error out"=w398:errorcluster, "RobotDriveDevRef"=w399:T6)  [unwired: 9 in]
              n158 = while {
                tunnel: w409 -> [w427]
                tunnel: w408 -> [w426]
                tunnel: w406 -> [w423]
                tunnel: w407 -> [w424]
                tunnel: [w420] -> w402
                tunnel: [w419] -> w401
                tunnel: [w418] -> _
                tunnel: [w417] -> _
                tunnel: [w416] -> w403
                tunnel: w399 -> [w415]
                tunnel: w398 -> [w414]
                stop <- w416 stop-if-true
                n159 = call <vilib>:"WPI_EncoderGet.vi"("error in (no error)"=w424, "EncoderDevRef"=w423) -> ("error out"=w417:errorcluster, "Distance"=→"Distance 25":dbl, "EncoderDevRef"=w418:T2)  [unwired: 4 in, 3 out]
                n160 = call <vilib>:"WPI_EncoderGet.vi"("error in (no error)"=w426, "EncoderDevRef"=w427) -> ("error out"=w419:errorcluster, "Distance"=w422:dbl, "EncoderDevRef"=w420:T2)  [unwired: 4 in, 3 out]
                "Distance 26" <- w422
                n161 = Greater Or Equal?(x=w422, y=5000.0) -> (x >= y?=w416:bool)
                n162 = call <vilib>:"WPI_RobotDriveMotors.vi"("error in (no error)"=w414, "RightSpeed"=0.5, "LeftSpeed"=0.5, "RobotDriveDevRef"=w415) -> ()  [unwired: 5 in, 3 out]
              }
              n163 = case shown="True" w403 {
                tunnel: w402 -> [_ w411]
                tunnel: w401 -> [_ w410]
                frame False {
                }
                frame True {
                  n164 = call <vilib>:"WPI_EncoderReset.vi"("error in (no error)"=w410, "EncoderDevRef"=w411) -> ()  [unwired: 8 in, 2 out]
                }
              }
            }
          }
        }
      }
    }
  }
